vi "vision state fg.vi"(2 "Action":T1, 3 "Menu":T2) -> (0 "State Out":T1, 1 "Enabled?":bool)   [LabVIEW 2014]
uses:
  typedefs/fg_getset.ctl
  typedefs/vision/vision enable.ctl
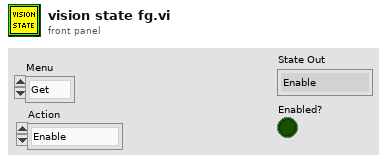
[diagram p1: front panel]
types:
  T1 = typedef "vision enable.ctl" = enum16{"Enable", "Disable", "Stop"}
  T2 = typedef "fg_getset.ctl" = enum16{"Get", "Set"}
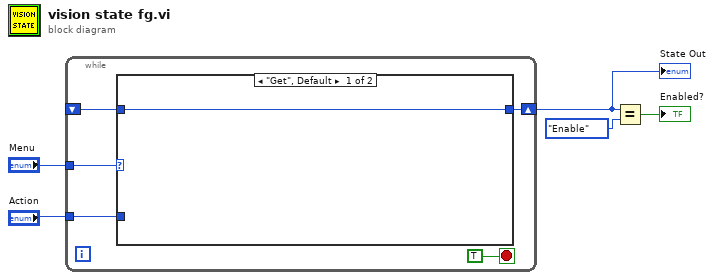
[diagram p0: block diagram]
diagram:
  n1 = while {
    shift-right: [w8] -> w4
    shift-left: _ -> [w9]
    tunnel: "Action" -> [w7]
    tunnel: "Menu" -> [w6]
    stop <- TRUE stop-if-true
    n2 = case shown="\"Get\", Default" w6 {
      tunnel: w9 -> [w11 _]
      tunnel: [w11 w12] -> w8
      tunnel: w7 -> [_ w12]
      frame "Get", Default {
      }
      frame "Set" {
      }
    }
  }
  "State Out" <- w4
  n3 = Equal?(x=w4, y=vision_enable."Enable") -> (x = y?=→"Enabled?":bool)
